vi "ClimbGlobals.vi"() -> ()   [LabVIEW 2020]
panel:
  in  "LeftClimbDemand":dbl
  in  "RightClimbDemand":dbl
  out "LeftLimit":bool
  out "RightLimit":bool
  in  "ClimbBackButton":bool
  out "Zero Request":bool
  out "ClimbOverride":bool
  in  "RightClimbEncoder":dbl
  in  "LeftClimbEncoder":dbl
  in  "ClimbSpeedDemand":dbl
  in  "ClimbButton":bool
  in  "ClimbState":i32
  in  "ArmForward":bool
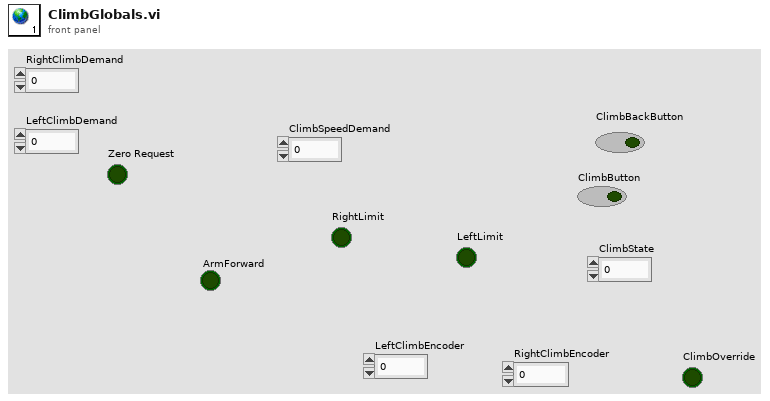
[diagram p1: front panel]
diagram:
